vi "TearingDown.vi"(6 "Error":errorcluster, 11 "Actor":refnum<class "Actor.lvclass">) -> (3 "Actor":refnum<class "Actor.lvclass">)   [LabVIEW 2020, in "jettl.lvlib"]
uses:
  jettl.lvlib
  Lifecycle.ctl
  Actor/Actor.lvclass
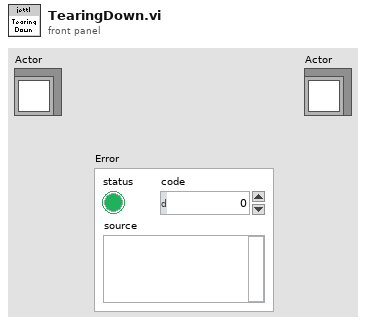
[diagram p1: front panel]
types:
  T1 = typedef "jettl.lvlib/Lifecycle.ctl" = enum16{"Initializing", "SettingUp", "TeardownBeforeStart", "Start", "Running", "Stop", "TeardownAfterStart"}
  T2 = typedef "jettl.lvlib/Base.ctl" = cluster{"Lifecycle":T3, "SelfActor":T4, "MediatorActor":T4, "ComponentActorMap":T9}
  T3 = typedef "jettl.lvlib/Lifecycle.ctl" = enum16{"Initializing", "SettingUp", "Starting", "Running", "Stopping", "TearingDown", "Terminated"}
  T4 = typedef "jettl.lvlib/Actor.ctl" = cluster{"Messages":T5, "ActorAlias":string, "ActorType":T8, "Transport":refnum<user-event>, "EventRegistrationRef":refnum<event-registration>, "VIRef":refnum<vi>}
  T5 = typedef "jettl.lvlib/Messages.ctl" = cluster{"Listen":T6, "TellSelf":T6, "TellMediator":T6, "TellComponentMap":T7}
  T6 = typedef "jettl.lvlib/MessageSet.ctl" = set{refnum<class "Message.lvclass">}
  T7 = typedef "jettl.lvlib/TellComponentMap.ctl" = map{string, T6}
  T8 = typedef "jettl.lvlib/ActorType.ctl" = enum16{"Mediator", "Component"}
  T9 = typedef "jettl.lvlib/ComponentActorMap.ctl" = map{string, T4}
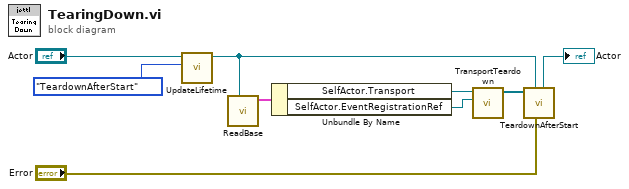
[diagram p0: block diagram]
diagram:
  n1 = call "UpdateLifetime.vi"("Lifecycle"=Lifecycle."TeardownAfterStart" ("Lifetime"), "Actor"="Actor") -> ("Actor"=w2:refnum<class "Actor.lvclass">)  [unwired: 9 in]
  n2 = call-dynamic "ReadBase.vi"("Actor"=w2) -> ("Base"=w8:T2)  [unwired: 10 in]
  n3 = Unbundle By Name(w8) -> ("SelfActor.Transport"=w7:refnum<user-event>, "SelfActor.EventRegistrationRef"=w6:refnum<event-registration>)
  n4 = call "TransportTeardown.vi"("EventRegistrationRef"=w6, "Transport"=w7) -> ("UnheardMessages"=w3:refnum<class "Message.lvclass">[])  [unwired: 9 in]
  n5 = call-dynamic "TeardownAfterStart.vi"("Error"="Error", "Actor"=w2, "UnheardMessages"=w3) -> ("Actor"=→"Actor":refnum<class "Actor.lvclass">)  [unwired: 8 in]
